vi "Get Type Names.vi"(8 "error in (no error)":errorcluster, 11 "Engine in":refnum<class "Engine.lvclass">) -> (0 "error out":errorcluster, 3 "Engine out":refnum<class "Engine.lvclass">)   [LabVIEW 2020, in "TSnax.lvlib" / "Engine.lvclass"]
uses:
  Engine.lvclass
  Engine.lvclass/Engine.ctl
  845e599d-73ce-492c-bb2f-ee1d946bdea8.vi
panel:
  out "Array":cluster{"TypeCategory":i32, "Name":string}[](array[cluster])
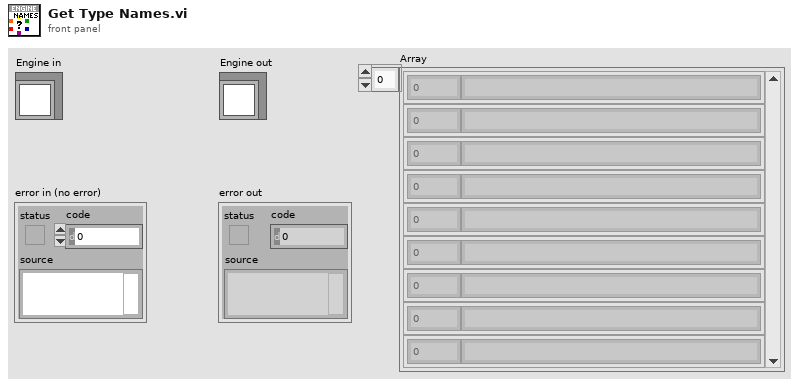
[diagram p1: front panel]
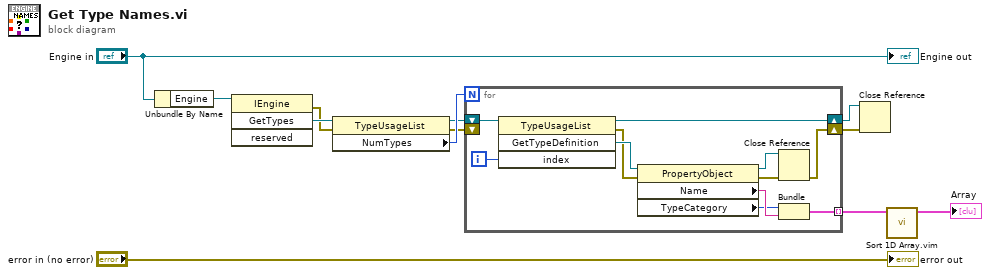
[diagram p0: block diagram]
diagram:
  n1 = Unbundle By Name("Engine in") -> ("Engine"=w10:refnum<k7>)
  n2 = invoke class="IEngine" method="GetTypes"(reference=w10) -> (error out=w6:errorcluster, "GetTypes"=w9:refnum<k7>)  [unwired: 3 in, 2 out]
  n3 = property class="TypeUsageList"(reference=w9, error in=w6) -> (reference out=w7:refnum<k7>, error out=w5:errorcluster, "NumTypes"=w8:i32)
  n4 = for {
    N: w8 -> [_]
    shift-right: [w21] -> w3
    shift-left: w7 -> [w23]
    shift-right: [w14] -> w4
    shift-left: w5 -> [_]
    tunnel: [w13] -> w2 mode=indexing
    i -> [w22]
    n5 = invoke class="TypeUsageList" method="GetTypeDefinition"(reference=w23, "index"=w22) -> (reference out=w21:refnum<k7>, error out=w15:errorcluster, "GetTypeDefinition"=w20:refnum<k7>)  [unwired: 2 in, 1 out]
    n6 = property class="PropertyObject"(reference=w20, error in=w15) -> (reference out=w16:refnum<k7>, error out=w17:errorcluster, "Name"=w19:string, "TypeCategory"=w18:i32)
    n7 = Close Reference(reference=w16, error in (no error)=w17) -> (error out=w14:errorcluster)
    n8 = Bundle("TypeCategory"=w18, "Name"=w19) -> (w13:cluster{"TypeCategory":i32, "Name":string})  [unwired: 1 in]
  }
  n9 = Close Reference(reference=w3, error in (no error)=w4) -> ()  [unwired: 1 out]
  n10 = call "Sort 1D Array.vim"("unsorted array"=w2) -> ("sorted array"=→"Array":cluster{"TypeCategory":i32, "Name":string}[])  [unwired: 10 in]
  "error out" <- "error in (no error)"
  "Engine out" <- "Engine in"
